vi "test24-MappingRelationshipByExternalRegistration_API.vi"(8 "error in (no error)":errorcluster, 11 "TestCase in":refnum<class "testcase-CSMBroadcast.lvclass">) -> (0 "error out":errorcluster, 3 "TestCase out":refnum<class "testcase-CSMBroadcast.lvclass">)   [LabVIEW 2017, in "testcase-CSMBroadcast.lvclass"]
uses:
  testcase-CSMBroadcast.lvclass
  src/user.lib/_NEVSTOP/Communicable State Machine(CSM)/Communicable State Machine.lvlib
  <vilib>/addons/_JKI Toolkits/VI Tester/TestCase.llb/TestCase.lvclass
  C:/Program Files (x86)/National Instruments/LabVIEW 2017/vi.lib/addons/_JKI Toolkits/VI Tester/TestCase.llb/TestCase.lvclass
panel:
  out "Loop Count":i32
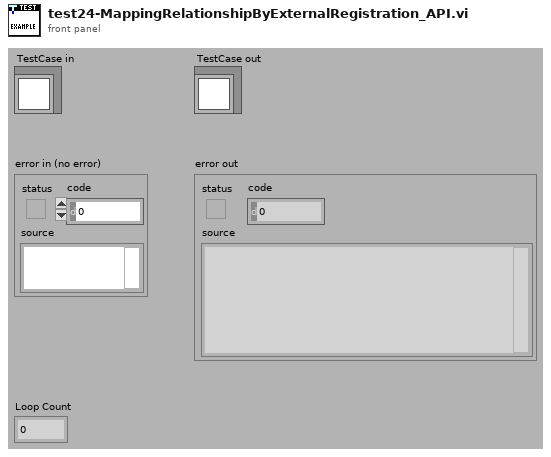
[diagram p1: front panel]
types:
  T1 = cluster{"Status":string, "Source CSM":string, "Target CSM":string, "Target API":string}[]
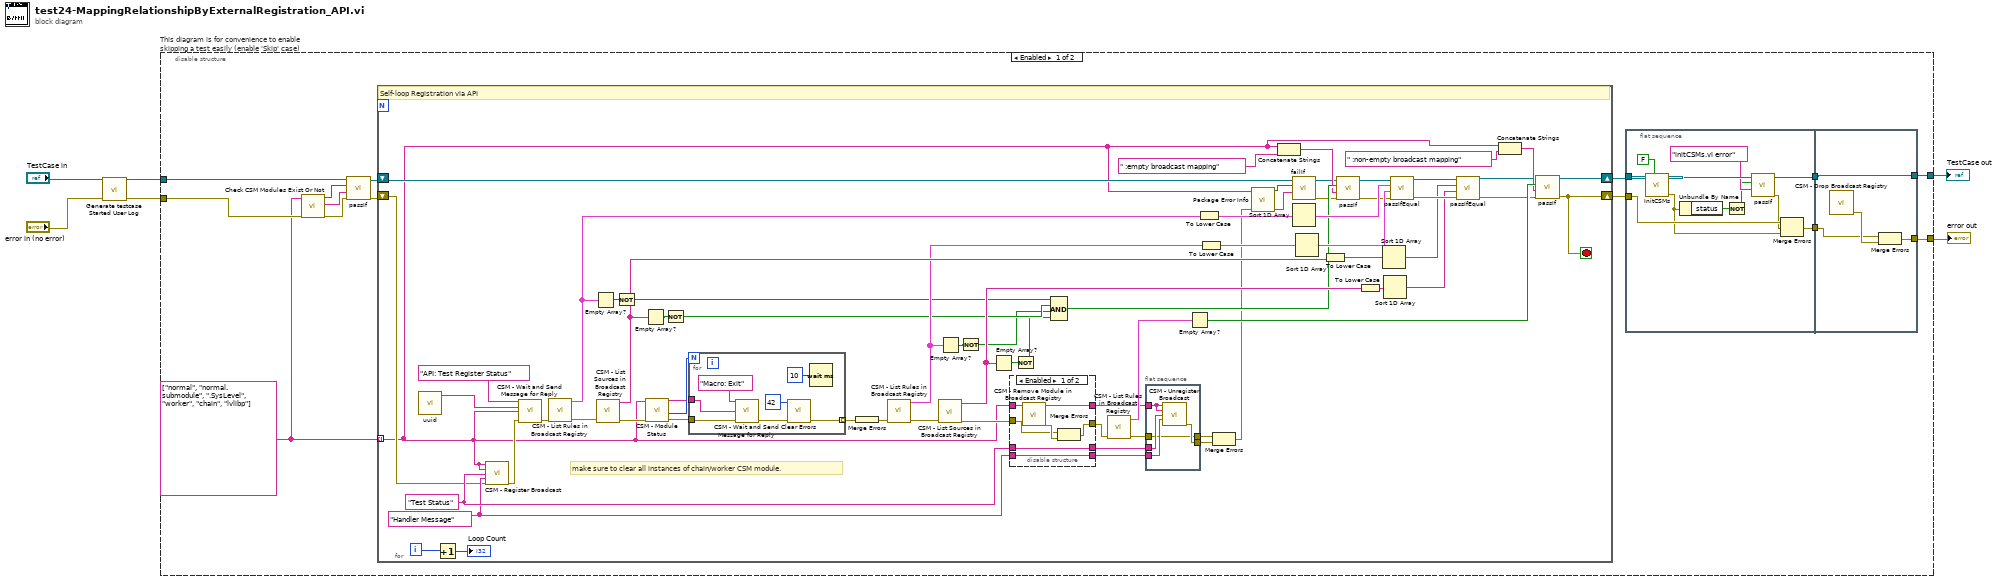
[diagram p0: block diagram]
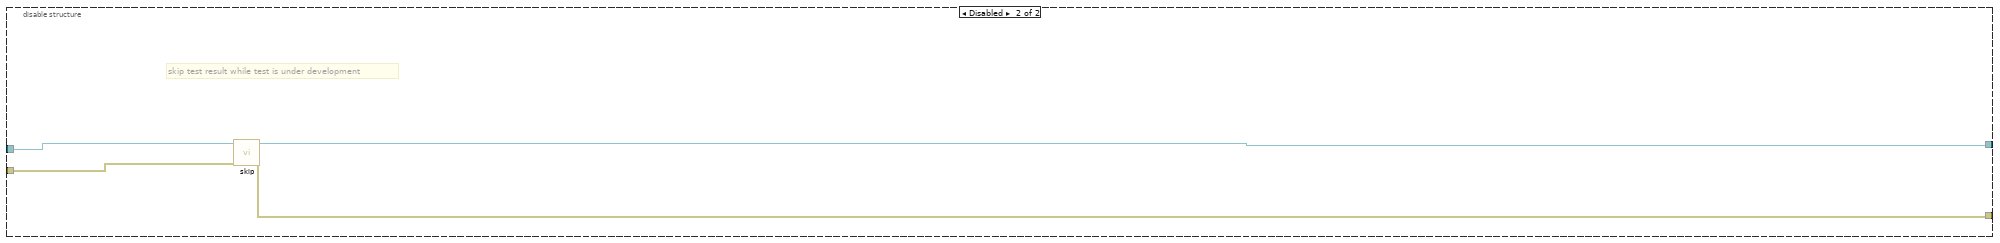
[diagram p3: hidden frame]
diagram:
  n1 = call "Generate testcase Started User Log.vi"("Error In"="error in (no error)") -> ("error out"=w1:errorcluster)  [unwired: 10 in]
  n2 = disable-structure "This diagram is for convenience to enable skipping a test easily (enable 'Skip' case)" shown="Enabled" {
    disable-tunnel: "TestCase in" -> [w13 w128]
    disable-tunnel: [w8 w126] -> w2
    disable-tunnel: [w7 w127] -> w4
    disable-tunnel: w1 -> [w11 w125]
    frame Enabled {
      w9 = string[] ["normal", "normal.submodule", ".SysLevel", "worker", "chain", "lvlibp"]
      n3 = call "Check CSM Modules Exist Or Not.vi"("error in"=w11, "CSM names in"=w9) -> ("error out"=w14:errorcluster, "Debug string"=w15:string, "All Modules Exist?"=w16:bool)  [unwired: 7 in]
      n4 = call-dynamic "passIf.vi"("error in (no error)"=w14, "message (\"\")"=w15, "pass"=w16, "TestCase in"=w13) -> ("error out"=w10:errorcluster, "TestCase out"=w12:refnum<class "testcase-CSMBroadcast.lvclass">)  [unwired: 6 in]
      n5 = for {
        tunnel: w9 -> [w43] mode=indexing
        shift-right: [w67] -> w18
        shift-left: w12 -> [w46]
        shift-right: [w65] -> w17
        shift-left: w10 -> [w53]
        i -> [w86]
        stop <- w65 stop-if-true
        w69 = "Handler Message" ("Response Message (If \"\", Same as Source Message)")
        w70 = "Test Status" ("Status")
        # "make sure to clear all instances of chain/worker CSM module."
        # "Self-loop Registration via API"
        n6 = call "uuid.vi"() -> ("UUID"=w100:string)  [unwired: 11 in]
        n7 = Increment(x=w86) -> (x+1=→"Loop Count":i32)
        n8 = call "CSM - Register Broadcast.vi"("CSM Name(Empty for Broadcast Event)"=w43, "Source CSM Name (* as Default)"=w43, "Trigger"=w70, "API (If \"\", Same as Trigger)"=w69, "Error In"=w53) -> ("error out"=w71:errorcluster)  [unwired: 9 in, 1 out]
        n9 = call "CSM - Wait and Send Message for Reply.vi"("State"="API: Test Register Status", "Arguments (\"\")"=w100, "Target Module"=w43, "Error In (No Error)"=w71) -> ("error out"=w99:errorcluster)  [unwired: 8 in, 3 out]
        n10 = call "CSM - List Rules in Broadcast Registry.vi"("error in (no error)"=w99) -> ("error out"=w98:errorcluster, "Rule Entries"=w84:T1)  [unwired: 8 in, 1 out]
        n11 = Empty Array?(array=w84) -> (empty?=w83:bool)
        n12 = call "CSM - List Sources in Broadcast Registry.vi"("error in (no error)"=w98) -> ("error out"=w62:errorcluster, "Broadcast Names"=w81:string[])  [unwired: 9 in]
        n13 = Not(x=w83) -> (.not. x?=w76:bool)
        n14 = Empty Array?(array=w81) -> (empty?=w82:bool)
        n15 = call "CSM - Module Status.vi"("Error In"=w62, "CSM Name"=w43) -> ("error out"=w61:errorcluster, "#Nodes"=w64:i32, "CSM Name (Dup)"=w63:string)  [unwired: 5 in, 2 out]
        n16 = Not(x=w82) -> (.not. x?=w75:bool)
        n17 = for {
          N: w64 -> [_]
          tunnel: w63 -> [w112]
          tunnel: w61 -> [w111]
          tunnel: [w109] -> w59 mode=indexing
          n18 = call "CSM - Wait and Send Message for Reply.vi"("State"="Macro: Exit", "Target Module"=w112, "Error In (No Error)"=w111) -> ("error out"=w110:errorcluster)  [unwired: 9 in, 3 out]
          n19 = call <vilib>:"Clear Errors.vi"("error in (no error)"=w110, "specific error code to clear (0: all)"=42) -> ("error out"=w109:errorcluster)  [unwired: 4 in, 1 out]
          n20 = Wait (ms)(milliseconds to wait=u32 10) -> ()  [unwired: 1 out]
        }
        n21 = Merge Errors(w59) -> (w60:errorcluster)
        n22 = call "CSM - List Rules in Broadcast Registry.vi"("error in (no error)"=w60) -> ("error out"=w97:errorcluster, "Rule Entries"=w79:T1)  [unwired: 8 in, 1 out]
        n23 = call "CSM - List Sources in Broadcast Registry.vi"("error in (no error)"=w97) -> ("error out"=w72:errorcluster, "Broadcast Names"=w77:string[])  [unwired: 9 in]
        n24 = Empty Array?(array=w79) -> (empty?=w80:bool)
        n25 = Not(x=w80) -> (.not. x?=w74:bool)
        n26 = Empty Array?(array=w77) -> (empty?=w78:bool)
        n27 = disable-structure shown="Enabled" {
          disable-tunnel: w72 -> [w114 w123]
          disable-tunnel: [w118 w123] -> w41
          disable-tunnel: w43 -> [w119 w124]
          disable-tunnel: w70 -> [w116 w122]
          disable-tunnel: w69 -> [w115 w121]
          disable-tunnel: [w117 w124] -> w42
          disable-tunnel: [w116 w122] -> w40
          disable-tunnel: [w115 w121] -> w39
          frame Enabled {
            n28 = call "CSM - Remove Module in Broadcast Registry.vi"("CSM Name"=w119) -> ("CSM Name (Dup)"=w117:string, "error out"=w120:errorcluster)  [unwired: 13 in]
            n29 = Merge Errors(w114, w120) -> (w118:errorcluster)
          }
          frame Disabled {
          }
        }
        n30 = Not(x=w78) -> (.not. x?=w73:bool)
        n31 = Compound Arithmetic op=AND(w76, w75, w74, w73) -> (w52:bool)
        n32 = call "CSM - List Rules in Broadcast Registry.vi"("error in (no error)"=w41) -> ("error out"=w36:errorcluster, "Rule Entries"=w68:T1)  [unwired: 8 in, 1 out]
        n33 = flat-sequence {
          tunnel: w42 -> [w106]
          tunnel: w40 -> [w105]
          tunnel: w39 -> [w104]
          tunnel: [w103] -> w38
          tunnel: w36 -> [w102]
          tunnel: [w102] -> w35
          frame #0 {
            n34 = call "CSM - Unregister Broadcast.vi"("CSM Name(Empty for Broadcast Event)"=w106, "Source CSM Name (* as Default)"=w106, "Trigger"=w105, "API (\"*\" as Default)"=w104) -> ("error out"=w103:errorcluster)  [unwired: 10 in, 1 out]
          }
        }
        n35 = Empty Array?(array=w68) -> (empty?=w66:bool)
        n36 = To Lower Case(string=w84) -> (all lower case string=w96:T1)
        n37 = To Lower Case(string=w79) -> (all lower case string=w95:T1)
        n38 = Merge Errors(w35, w38) -> (w37:errorcluster)
        n39 = call "Package Error Info.vi"("error in"=w37, "String in"=w43) -> ("packed error info out"=w47:string, "error status"=w48:bool)  [unwired: 8 in]
        n40 = Concatenate Strings(w43, " :empty broadcast mapping" ("string")) -> (w51:string)
        n41 = call-dynamic "failIf.vi"("message (\"\")"=w47, "fail"=w48, "TestCase in"=w46) -> ("error out"=w44:errorcluster, "TestCase out"=w45:refnum<class "testcase-CSMBroadcast.lvclass">)  [unwired: 7 in]
        n42 = Sort 1D Array(array=w96) -> (sorted array=w94:T1)
        n43 = Sort 1D Array(array=w95) -> (sorted array=w93:T1)
        n44 = To Lower Case(string=w81) -> (all lower case string=w90:string[])
        n45 = call-dynamic "passIf.vi"("error in (no error)"=w44, "message (\"\")"=w51, "pass"=w52, "TestCase in"=w45) -> ("error out"=w55:errorcluster, "TestCase out"=w54:refnum<class "testcase-CSMBroadcast.lvclass">)  [unwired: 6 in]
        n46 = To Lower Case(string=w77) -> (all lower case string=w89:string[])
        n47 = Sort 1D Array(array=w90) -> (sorted array=w88:string[])
        n48 = Sort 1D Array(array=w89) -> (sorted array=w87:string[])
        n49 = call-dynamic "passIfEqual.vi"("error in (no error)"=w55, "y"=w93, "x"=w94, "TestCase in"=w54) -> ("error out"=w91:errorcluster, "TestCase out"=w92:refnum<class "testcase-CSMBroadcast.lvclass">)  [unwired: 6 in]
        n50 = call-dynamic "passIfEqual.vi"("error in (no error)"=w91, "y"=w87, "x"=w88, "TestCase in"=w92) -> ("error out"=w49:errorcluster, "TestCase out"=w50:refnum<class "testcase-CSMBroadcast.lvclass">)  [unwired: 6 in]
        n51 = Concatenate Strings(w43, " :non-empty broadcast mapping" ("string")) -> (w56:string)
        n52 = call-dynamic "passIf.vi"("error in (no error)"=w49, "message (\"\")"=w56, "pass"=w66, "TestCase in"=w50) -> ("error out"=w65:errorcluster, "TestCase out"=w67:refnum<class "testcase-CSMBroadcast.lvclass">)  [unwired: 6 in]
      }
      n53 = flat-sequence {
        tunnel: w18 -> [w30]
        tunnel: [w27] -> w19
        tunnel: w17 -> [w24]
        tunnel: [w21] -> w6
        tunnel: w19 -> [w33]
        tunnel: [w33] -> w8
        tunnel: [w32] -> w7
        tunnel: w6 -> [w31]
        frame #0 {
          n54 = call "InitCSMs.vi"("Enable building lvlibp?"=FALSE, "testcase-CSMStatus in"=w30) -> ("error out"=w22:errorcluster, "testcase-CSMStatus out"=w28:refnum<class "testcase-CSMBroadcast.lvclass">)  [unwired: 8 in]
          n55 = Unbundle By Name(w22) -> ("status"=w26:bool)
          n56 = Not(x=w26) -> (.not. x?=w20:bool)
          n57 = call-dynamic "passIf.vi"("message (\"\")"="initCSMs.vi error" ("message (\"\")"), "pass"=w20, "TestCase in"=w28) -> ("error out"=w23:errorcluster, "TestCase out"=w27:refnum<class "testcase-CSMBroadcast.lvclass">)  [unwired: 7 in]
          n58 = Merge Errors(w24, w23, w22) -> (w21:errorcluster)
        }
        frame #1 {
          n59 = call "CSM - Drop Broadcast Registry.vi"() -> ("error out"=w34:errorcluster)  [unwired: 15 in]
          n60 = Merge Errors(w31, w34) -> (w32:errorcluster)
        }
      }
    }
    frame Disabled {
      # "skip test result while test is under development"
      n61 = call <vilib>:"skip.vi"("error in (no error)"=w125, "TestCase in"=w128) -> ("error out"=w127:errorcluster, "TestCase out"=w126:refnum<class "testcase-CSMBroadcast.lvclass">)  [unwired: 8 in]
    }
  }
  "error out" <- w4
  "TestCase out" <- w2
